vi "Force Props.vi"(8 "error in (no error)":errorcluster, 11 "Board Info for checking":T1) -> (0 "error out":errorcluster, 2 "scaling info out":variant, 3 "bridge info out":variant)   [LabVIEW 2010, in "PXIe-433x Custom Device.lvlib"]
uses:
  PXIe-433x Custom Device.lvlib
  Max Value.ctl
  Min Value.ctl
  Generic Bridge Information.ctl
  Force Scaling Information.ctl
  Board Info for checking settings.ctl
  Scale Type.ctl
  Sensor Type.ctl
panel:
  in  "physical units":i32(ring)=15876 items=["Newtons"=15875, "Pounds"=15876, "kgf"=15877]
  in  "scaling information":T2={"first electrical value"=0.0, "second electrical value"=2.0, "electrical units"=15897, "first physical value"=0.0, "second physical value"=100.0, "physical units"=15876} {"physical units" items=["Newtons"=15875, "Pounds"=15876, "kgf"=15877]; "electrical units" items=["Volts/Volt"=15896, "mVolts/Volt"=15897]}
  in  "bridge information":T3={"bridge configuration"=10182, "voltage excitation source"=10200, "voltage excitation value"=2.5, "nominal bridge resistance"=350.0} {"voltage excitation source" items=["Internal"=10200, "External"=10167]; "bridge configuration" items=["Full Bridge"=10182, "Half Bridge"=10187, "Quarter Bridge"=10270]}
  in  "Minimum Value":T4=-5000.0 caption="Pounds"
  in  "Maximum Value":T5=5000.0 caption="Pounds"
  out "Error Description":string
  out "Tab Control":enum32{"No Error", "No Check", "Error"}(tab)
  out "Valid":bool=TRUE
  in  "No Error Check Details":bool
  out "No Check":bool=TRUE
  in  "Error Details":bool
  in  "stop":bool
  out "Valid Configuration?":bool
  # "No Error"
  # "No Error"
  # "No Error Check"
  # "No Error Check"
  # "Error!"
  # "Error!"
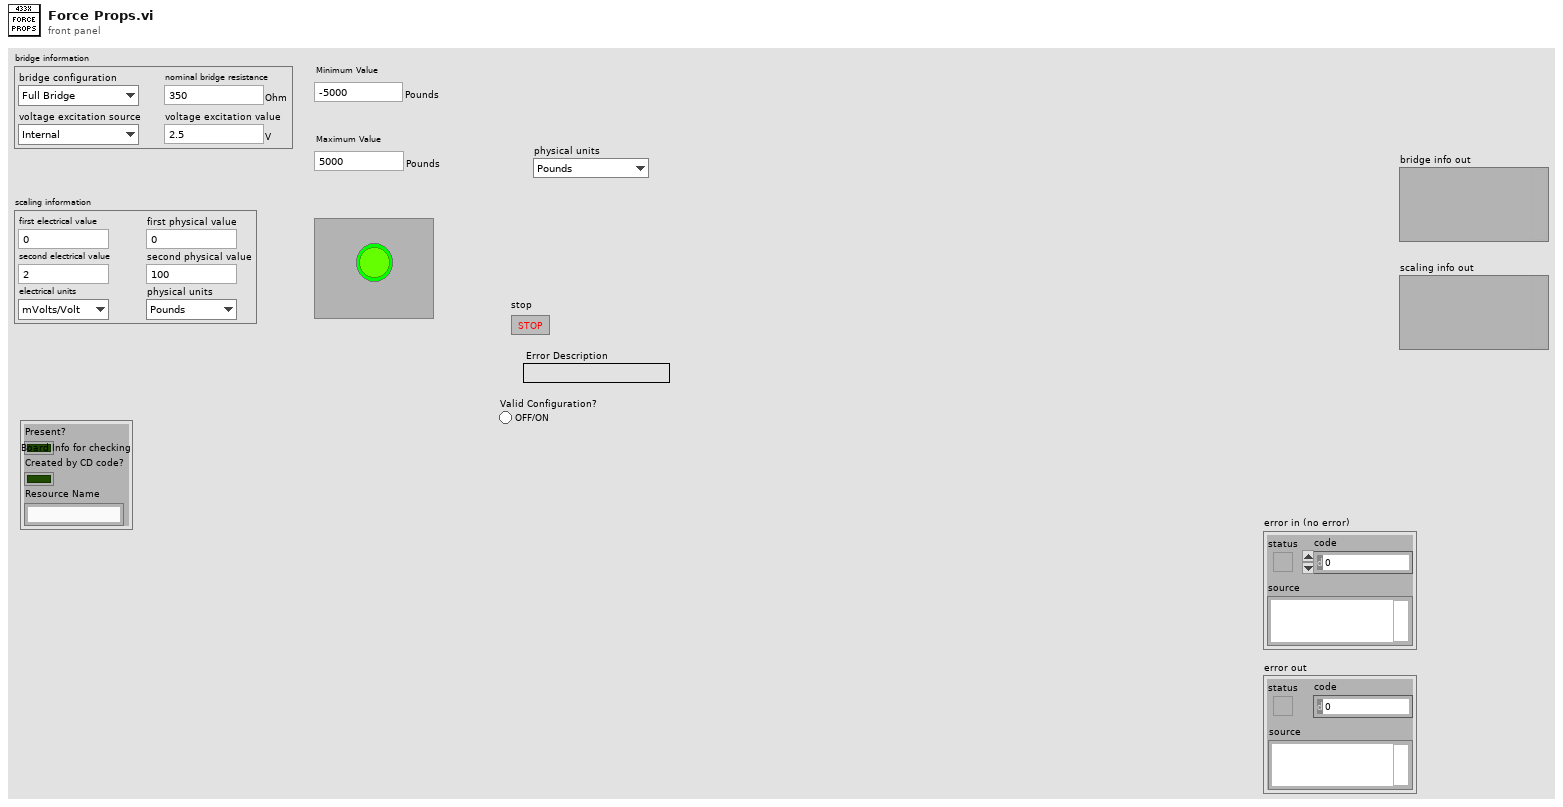
[diagram p1: front panel]
types:
  T1 = typedef "PXIe-433x Custom Device.lvlib/Board Info for checking settings.ctl" = cluster{"Present?":bool, "Created by CD code?":bool, "Resource Name":string}
  T2 = typedef "PXIe-433x Custom Device.lvlib/Force Scaling Information.ctl" = cluster{"first electrical value":dbl, "second electrical value":dbl, "electrical units":i32, "first physical value":dbl, "second physical value":dbl, "physical units":i32}
  T3 = typedef "PXIe-433x Custom Device.lvlib/Generic Bridge Information.ctl" = cluster{"bridge configuration":i32, "voltage excitation source":i32, "voltage excitation value":dbl, "nominal bridge resistance":dbl}
  T4 = typedef "PXIe-433x Custom Device.lvlib/Min Value.ctl" = dbl
  T5 = typedef "PXIe-433x Custom Device.lvlib/Max Value.ctl" = dbl
  T6 = typedef "PXIe-433x Custom Device.lvlib/Scale Type.ctl" = enum16{"Linear", "Table", "Polynomial"}
  T7 = typedef "PXIe-433x Custom Device.lvlib/Sensor Type.ctl" = enum16{"Strain", "Force", "Pressure", "Torque"}
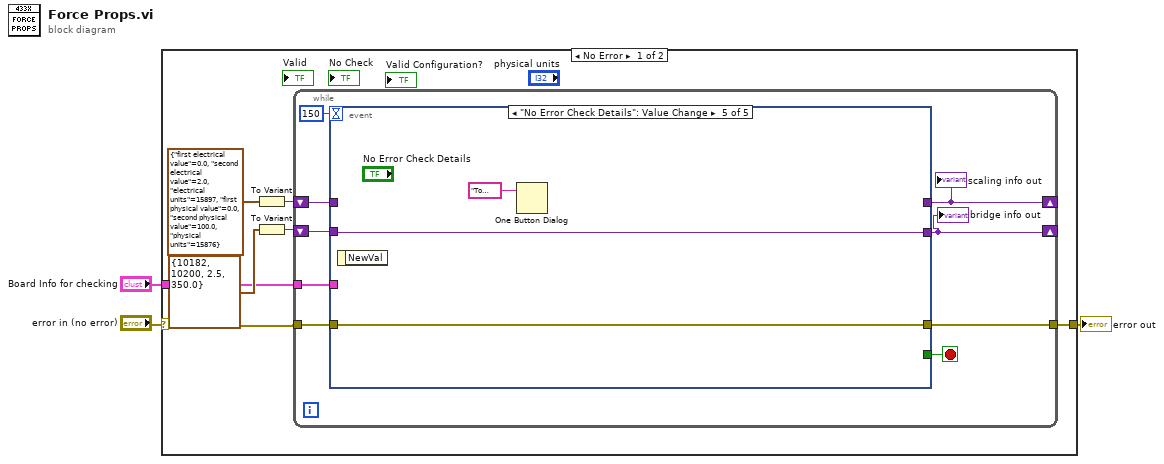
[diagram p0: block diagram]
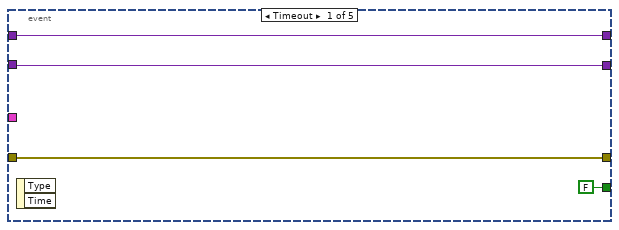
[diagram p2: hidden frame]
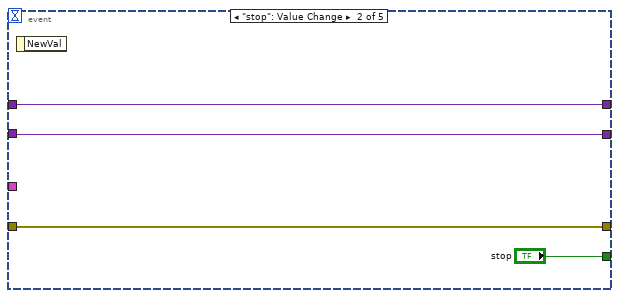
[diagram p3: hidden frame]
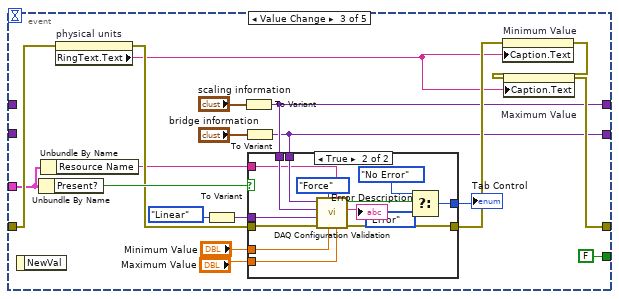
[diagram p4: hidden frame]
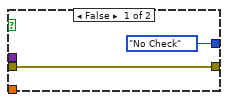
[diagram p5: hidden frame]
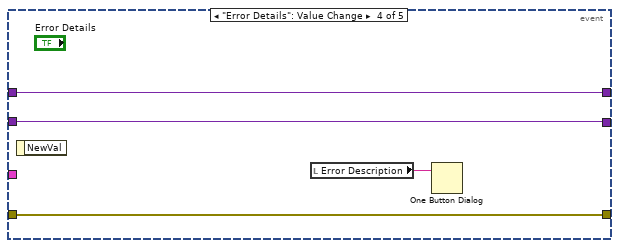
[diagram p6: hidden frame]
diagram:
  n1 = case shown="No Error" "error in (no error)" {
    selector: "error in (no error)" -> [w5 w70]
    tunnel: [w10 w70] -> w2
    tunnel: "Board Info for checking" -> [w4 _]
    frame No Error {
      n2 = To Variant(anything=T2 {"first electrical value"=0.0, "second electrical value"=2.0, "electrical units"=15897, "first physical value"=0.0, "second physical value"=100.0, "physical units"=15876} ("scaling information")) -> (Variant=w9:variant)
      n3 = To Variant(anything=T3 {"bridge configuration"=10182, "voltage excitation source"=10200, "voltage excitation value"=2.5, "nominal bridge resistance"=350.0} ("bridge information")) -> (Variant=w8:variant)
      n4 = while {
        tunnel: w5 -> [w19]
        tunnel: [w17] -> w10
        shift-right: [w15] -> _
        shift-left: w9 -> [w12]
        shift-right: [w14] -> _
        shift-left: w8 -> [w13]
        tunnel: w4 -> [w11]
        stop <- w18 stop-if-true
        n5 = event shown="[4] \"No Error Check Details\": Value Change" {
          selector: _ -> [_ _ _ _ _]
          dyn-events: _ -> [_ _ _ _ _]
          timeout: 150 -> [_ _ _ _ _]
          tunnel: w19 -> [w22 w26 w34 w66 w69]
          tunnel: [FALSE ("stop") "stop" FALSE ("stop") _ _] -> w18
          tunnel: [w22 w26 w36 w66 w69] -> w17
          tunnel: [w21 w25 w31 w64 _] -> w15
          tunnel: [w20 w24 w30 w63 w68] -> w14
          tunnel: w13 -> [w20 w24 _ w63 w68]
          tunnel: w12 -> [w21 w25 _ w64 _]
          tunnel: w11 -> [_ _ w29 _ _]
          event Timeout {
            n6 = event-data() -> ()  [unwired: 1 in, 2 out]
          }
          event "stop": Value Change {
            n7 = event-data() -> ()  [unwired: 1 in, 1 out]
          }
          event Value Change {
            n8 = event-data() -> ()  [unwired: 1 in, 1 out]
            n9 = Unbundle By Name(w29) -> ("Present?"=w46:bool)
            n10 = Unbundle By Name(w29) -> ("Resource Name"=w28:string)
            n11 = property on="physical units" class="Ring (strict)"(error in=w34) -> (error out=w33:errorcluster, "RingText.Text"=w32:string)  [unwired: 1 in, 1 out]
            n12 = To Variant(anything=Scale_Type."Linear" ("Scale Type")) -> (Variant=w40:variant)
            n13 = To Variant(anything="scaling information") -> (Variant=w31:variant)
            n14 = To Variant(anything="bridge information") -> (Variant=w30:variant)
            n15 = case shown="True" w46 {
              tunnel: w33 -> [w48 w62]
              tunnel: [w48 w55] -> w38
              tunnel: "Minimum Value" -> [_ w60]
              tunnel: "Maximum Value" -> [_ w59]
              tunnel: w31 -> [_ w57]
              tunnel: w30 -> [_ w58]
              tunnel: [enum32{"No Error", "No Check", "Error"}."No Check" ("Tab Control") w53] -> w41
              tunnel: w40 -> [_ w50]
              tunnel: w28 -> [_ w49]
              frame False {
              }
              frame True {
                n16 = call "DAQ Configuration Validation.vi"("Maximum Value"=w59, "DAQ Resource Name"=w49, "Minimum Value"=w60, "Sensor Type"=Sensor_Type."Force", "error in"=w62, "scale type"=w50, "scaling info"=w57, "bridge info"=w58) -> ("error IO"=w55:errorcluster, "Error Source"=→"Error Description":string, "Valid configuration?"=w51:bool)  [unwired: 1 in]
                n17 = Select(t=enum32{"No Error", "No Check", "Error"}."No Error" ("Tab Control"), s=w51, f=enum32{"No Error", "No Check", "Error"}."Error" ("Tab Control")) -> (s? t:f=w53:enum32{"No Error", "No Check", "Error"})
              }
            }
            "Tab Control" <- w41
            n18 = property on="Minimum Value" class="DigNum (strict)"(error in=w38, "Caption.Text"=w32) -> (error out=w37:errorcluster)  [unwired: 1 in, 1 out]
            n19 = property on="Maximum Value" class="DigNum (strict)"(error in=w37, "Caption.Text"=w32) -> (error out=w36:errorcluster)  [unwired: 1 in, 1 out]
          }
          event "Error Details": Value Change {
            n20 = event-data() -> ()  [unwired: 1 in, 1 out]
            n21 = local read "Error Description"() -> (w65:string)
            n22 = One Button Dialog(message=w65) -> ()  [unwired: 1 in, 1 out]
          }
          event "No Error Check Details": Value Change {
            n23 = event-data() -> ()  [unwired: 1 in, 1 out]
            n24 = One Button Dialog(message="To perform error checking during Edition time, code needs either a physical local PXIe-433x or simulated one. One simulated couldn't be created, no error checking will be performed while editing settings. Error checking will still be performed while deploying Custom-Device.") -> ()  [unwired: 1 in, 1 out]
          }
        }
        "scaling info out" <- w15
        "bridge info out" <- w14
      }
    }
    frame Error {
    }
  }
  "error out" <- w2
